vi "Update Sub Panel.vi"(8 "error in (no error)":errorcluster, 9 "UI Section":string, 10 "Clone Name":string, 11 "UI Main in":refnum<class "UI Main.lvclass">) -> (0 "error out":errorcluster, 3 "UI Main out":refnum<class "UI Main.lvclass">)   [LabVIEW 2020, in "UI Main.lvlib" / "UI Main.lvclass"]
doc: "Send user event to update the sub panel."
uses:
  UI Main.lvclass
  Sub Panel.ctl
  UI Main.lvclass/UI Main.ctl
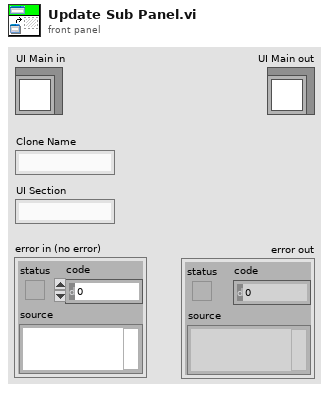
[diagram p1: front panel]
types:
  T1 = typedef "UI Main.lvlib/UI Main.lvclass/Sub Panel.ctl" = cluster{"Clone Name":string, "UI Section":string}
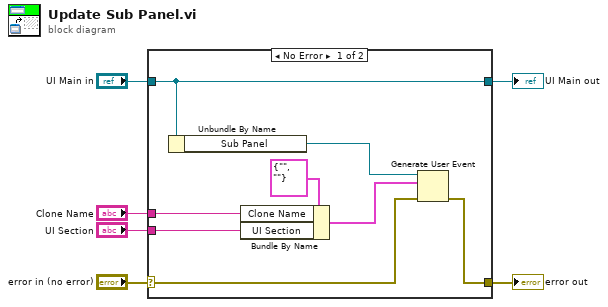
[diagram p0: block diagram]
diagram:
  n1 = case shown="No Error" "error in (no error)" {
    selector: "error in (no error)" -> [w10 w16]
    tunnel: [w9 w16] -> w5
    tunnel: [w14 w15] -> w3
    tunnel: "UI Main in" -> [w14 w15]
    tunnel: "Clone Name" -> [w8 _]
    tunnel: "UI Section" -> [w7 _]
    frame No Error {
      n2 = Unbundle By Name(w14) -> ("Sub Panel"=w13:refnum<user-event>)
      n3 = Bundle By Name(cluster=T1 {"Clone Name"="", "UI Section"=""} ("Sub Panel"), "Clone Name"=w8, "UI Section"=w7) -> (w11:T1)
      n4 = Generate User Event(user event=w13, event data cluster=w11, error in=w10) -> (error out=w9:errorcluster)  [unwired: 1 in, 1 out]
    }
    frame Error {
    }
  }
  "error out" <- w5
  "UI Main out" <- w3
